vi "Rohde & Schwarz VNA Set IFBW.vi"(6 "Channel":i8=1 min=1 max=99 step=1, 7 "Rohde & Schwarz VNA":T1, 8 "error in (no error)":errorcluster, 10 "IFBW, Hz (3000)":dbl=3000.0, 11 "VISA Resource Name":refnum<visa-resource-name>) -> (0 "error out":errorcluster, 3 "dup VISA Resource Name":refnum<visa-resource-name>)   [LabVIEW 2011]
doc: "This Vi for the HP8753B Network Analyzer is used to set averaging, smoothing, and the IF bandwidth."
uses:
  TypeDefs/Rohde & Schwarz VNA Instrument Info.ctl
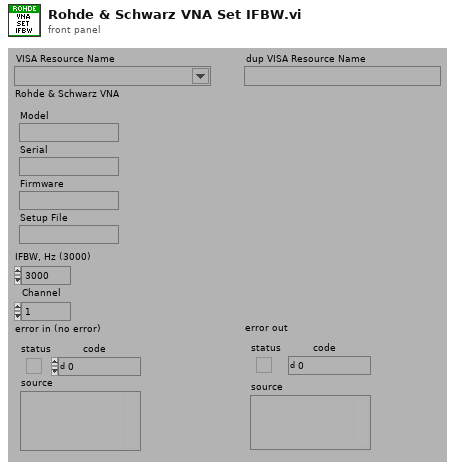
[diagram p1: front panel]
types:
  T1 = typedef "Rohde & Schwarz VNA Instrument Info.ctl" = cluster{"Model":string, "Serial":string, "Firmware":string, "Setup File":string}
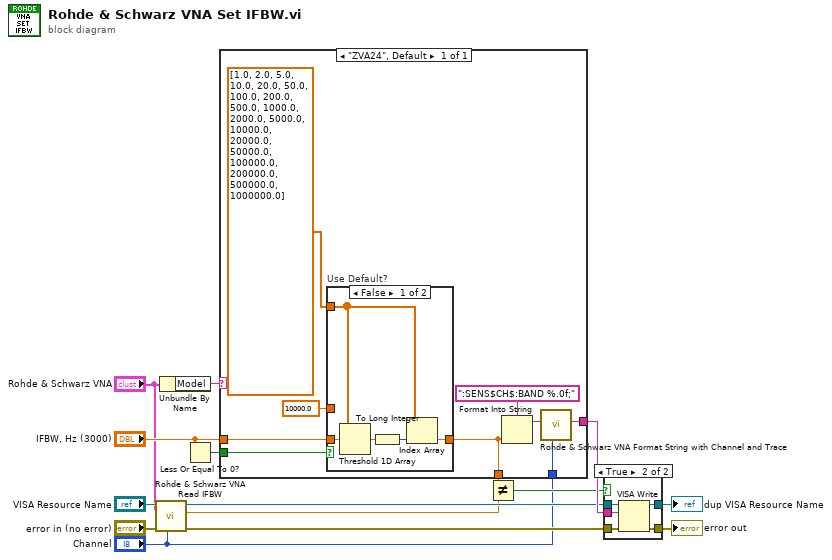
[diagram p0: block diagram]
diagram:
  n1 = call "Rohde & Schwarz VNA Read IFBW.vi"("Channel"="Channel", "Rohde & Schwarz VNA"="Rohde & Schwarz VNA", "error in (no error)"="error in (no error)", "VISA Resource Name"="VISA Resource Name") -> ("error out"=w9:errorcluster, "IFBW, Hz"=w7:dbl, "dup VISA Resource Name"=w10:refnum<visa-resource-name>)  [unwired: 5 out]
  n2 = Unbundle By Name("Rohde & Schwarz VNA") -> ("Model"=w1:string)
  n3 = Less Or Equal To 0?(x="IFBW, Hz (3000)") -> (x <= 0?=w4:bool)
  n4 = case shown="\"ZVA24\", Default" w1 {
    tunnel: "IFBW, Hz (3000)" -> [w20]
    tunnel: [w17] -> w13
    tunnel: [w19] -> w6
    tunnel: w4 -> [w23]
    tunnel: "Channel" -> [w16]
    frame "ZVA24", Default {
      n5 = case "Use Default?" shown="False" w23 {
        tunnel: dbl[] [1.0, 2.0, 5.0, 10.0, 20.0, 50.0, 100.0, 200.0, 500.0, 1000.0, 2000.0, 5000.0, 10000.0, 20000.0, 50000.0, 100000.0, 200000.0, 500000.0, 1000000.0] -> [w28 _]
        tunnel: w20 -> [w26 _]
        tunnel: [w25 w30] -> w19
        tunnel: 10000.0 -> [_ w30]
        frame False {
          n6 = Threshold 1D Array(2:w26, 3:w28) -> (0:w29:dbl)  [unwired: 1 out]
          n7 = To Long Integer(number=w29) -> (32bit integer=w27:i32)
          n8 = Index Array(array=w28, index=w27) -> (element=w25:dbl)
        }
        frame True {
        }
      }
      n9 = Format Into String(format string=":SENS$CH$:BAND %.0f;", w19) -> (resulting string=w18:string)  [unwired: 2 in, 1 out]
      n10 = call "Rohde & Schwarz VNA Format String with Channel and Trace.vi"("Channel"=w16, "String"=w18) -> ("String Out"=w17:string)  [unwired: 1 in, 6 out]
    }
  }
  n11 = Not Equal?(x=w6, y=w7) -> (x != y?=w8:bool)
  n12 = case shown="True" w8 {
    tunnel: [w31 w37] -> w15
    tunnel: [w32 w36] -> w14
    tunnel: w13 -> [_ w35]
    tunnel: w10 -> [w32 w34]
    tunnel: w9 -> [w31 w33]
    frame False {
    }
    frame True {
      n13 = VISA Write(VISA resource name=w34, write buffer=w35, error in (no error)=w33) -> (VISA resource name out=w36:refnum<visa-resource-name>, error out=w37:errorcluster)  [unwired: 1 out]
    }
  }
  "error out" <- w15
  "dup VISA Resource Name" <- w14
